vi "读取-数据库操作.lvclass.vi"(8 "error in (no error)":errorcluster caption="错误输入（无错误）", 11 "Admin客户端输入":refnum<class "Admin客户端.lvclass">) -> (0 "error out":errorcluster caption="错误输出", 2 "数据库操作.lvclass":refnum<class "数据库操作.lvclass">, 3 "Admin客户端输出":refnum<class "Admin客户端.lvclass">)   [LabVIEW 2013, in "Admin客户端.lvclass"]
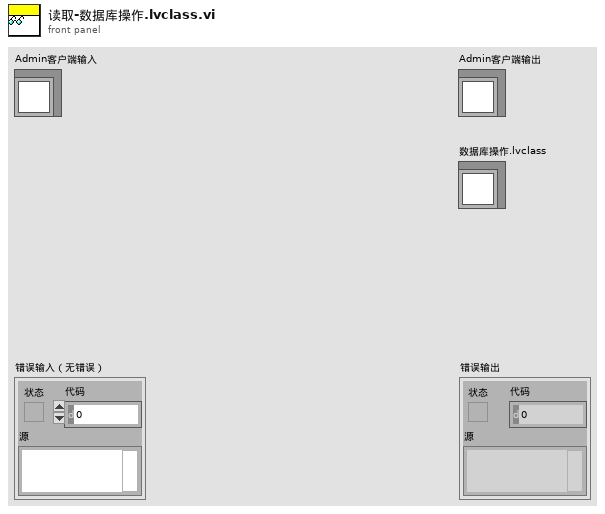
[diagram p1: front panel]
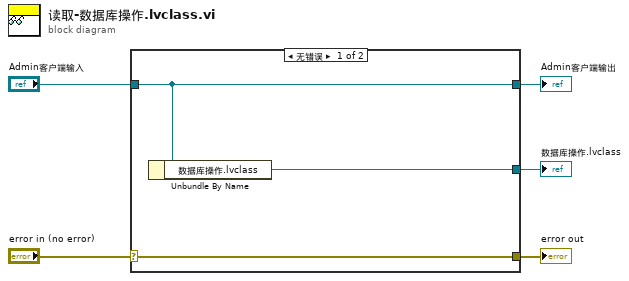
[diagram p0: block diagram]
diagram:
  n1 = case shown="无错误" "error in (no error)" {
    selector: "error in (no error)" -> [w8 w9]
    tunnel: [w8 w9] -> w4
    tunnel: [w7 w10] -> w2
    tunnel: "Admin客户端输入" -> [w7 w10]
    tunnel: [w6 _] -> w1
    frame No Error {
      n2 = Unbundle By Name(w7) -> ("数据库操作.lvclass"=w6:refnum<class "数据库操作.lvclass">)
    }
    frame Error {
    }
  }
  "error out" <- w4
  "Admin客户端输出" <- w2
  "数据库操作.lvclass" <- w1
